vi "mean and SD.vi"(11 "Input":dbl[](array[numeric])) -> (1 "skewness":dbl format="%0.2f", 2 "SD":dbl, 3 "mean":dbl)   [LabVIEW 2023]
uses:
  <vilib>/Analysis/baseanly.llb/Mean (DBL).vi
  <vilib>/Analysis/NI_AALBase.lvlib
  <vilib>/Analysis/NI_AALPro.lvlib
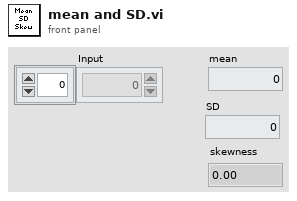
[diagram p1: front panel]
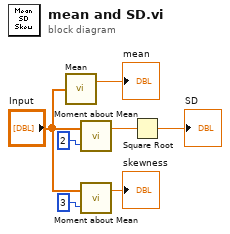
[diagram p0: block diagram]
diagram:
  n1 = call-poly <vilib>:"Mean.vi"("X"="Input") -> ("mean"=→"mean":dbl)  [unwired: 1 out]
  n2 = call <vilib>:"Moment about Mean.vi"("order"=2, "X"="Input") -> ("moment"=w5:dbl)  [unwired: 1 out]
  n3 = call <vilib>:"Moment about Mean.vi"("order"=3, "X"="Input") -> ("moment"=→"skewness":dbl)  [unwired: 1 out]
  n4 = Square Root(x=w5) -> (sqrt(x)=→"SD":dbl)
